vi "Elevator Offset AutoMatic.vi"() -> ()   [LabVIEW 2014]
uses:
  <vilib>/Rock Robotics/WPI/Joystick/WPI_JoystickGetSetRefNum.vi
panel:
  in  "Time Step(ms)":u32=10
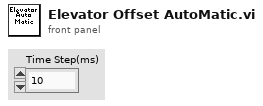
[diagram p1: front panel]
types:
  T1 = typedef "WPI_JoystickDevRef.ctl" = cluster{"Device":T2}
  T2 = typedef "WPI_JoystickDeviceEnum.ctl" = enum16{"USB 0", "USB 1", "USB 2", "USB 3", "USB 4", "USB 5"}
  T3 = typedef "WPI_MotorControlDeviceRef.ctl" = cluster{"DeviceStatus":errorcluster, "Type":T4, "PWM":cluster{"Controller":T5, "PWM Channel":T6, "DeadBand":T7}, "CAN":cluster{"Device Number":u8, "Control Mode":T8, "Semaphore":T9, "Max Vout":dbl, "TalonSRX Control Mode":T10}, "Invert":bool, "TransformRef":T11, "InvTransformRef":T11}
  T4 = typedef "WPI_MotorControlType.ctl" = enum16{"PWM", "CAN", "CANTalonSRX"}
  T5 = typedef "FPGA_TypedefDigitalModule.ctl" = enum16{"Controller 1"}
  T6 = typedef "FPGA_DIOPWMChannel.ctl" = enum8{"PWM 0", "PWM 1", "PWM 2", "PWM 3", "PWM 4", "PWM 5", "PWM 6", "PWM 7", "PWM 8", "PWM 9", "PWM MXP 0", "PWM MXP 1", "PWM MXP 2", "PWM MXP 3", "PWM MXP 4", "PWM MXP 5", "PWM MXP 6", "PWM MXP 7", "PWM MXP 8", "PWM MXP 9", "Invalid"}
  T7 = typedef "WPI_PWMDeadband.ctl" = cluster{"Name":string, "maxPositivePwm":i32, "minPositivePwm":i32, "centerPwm":i32, "maxNegativePwm":i32, "minNegativePwm":i32, "angularRange":u16}
  T8 = typedef "WPI_CANJaguar_ControlMode.ctl" = enum8{"Percent VBus", "Current", "Speed", "Position", "Voltage"}
  T9 = typedef "Semaphore RefNum" = refnum<k1>
  T10 = typedef "WPI_CANTalonSRX_APIControlMode.ctl" = enum8{"Percent VBus", "Speed", "Position", "Slave", "Unchanged / Invalid"}
  T11 = typedef "WPI_PWMTransform_ConPane.ctl" = refnum<vi>
  T12 = typedef "WPI_CANTalonSRX_GlobalStatus.ctl" = cluster{"Applied Throttle":dbl, "Module Enabled":bool, "CAN Error":errorcluster, "Closed Loop Error":dbl, "Forward Limit Switch Closed":bool, "Reverse Limit Switch Closed":bool, "Sensor Position":dbl, "Sensor Velocity":dbl, "Current":dbl, "Sticky Fault - Over Temp":bool, "Sticky Fault - Under Voltage":bool, "Sticky Fault - Forward Limit":bool, "Sticky Fault - Reverse Limit":bool, "Sticky Fault - Forward Soft Limit":bool, "Sticky Fault - Reverse Soft Limit":bool, "Brake is Enabled":bool, "Encoder Position":dbl, "Encoder Velocity":dbl, "Encoder Index Count":dbl, "Encoder A Pin State":bool, "Encoder B Pin State":bool, "Encoder Index Pin State":bool, "Analog In":dbl, "Analog In Velocity":dbl, "Temperature (C)":dbl, "Battery Voltage":dbl}
  T13 = typedef "WPI_SwitchDevRef.ctl" = cluster{"DevStatus":errorcluster, "DIO Channel":T14, "Controller":T5, "CntIndex":T15, "Normally Closed":bool}
  T14 = typedef "FPGA_DIOChannel.ctl" = enum8{"DIO 0", "DIO 1", "DIO 2", "DIO 3", "DIO 4", "DIO 5", "DIO 6", "DIO 7", "DIO 8", "DIO 9", "DIO MXP 0", "DIO MXP 1", "DIO MXP 2", "DIO MXP 3", "DIO MXP 4", "DIO MXP 5", "DIO MXP 6", "DIO MXP 7", "DIO MXP 8", "DIO MXP 9", "DIO MXP 10", "DIO MXP 11", "DIO MXP 12", "DIO MXP 13", "DIO MXP 14", "DIO MXP 15", "Invalid"}
  T15 = typedef "FPGA_CounterCtrSystemIndex.ctl" = enum8{"Ctr 0", "Ctr 1", "Ctr 2", "Ctr 3", "Ctr 4", "Ctr 5", "Ctr 6", "Ctr 7", "Invalid"}
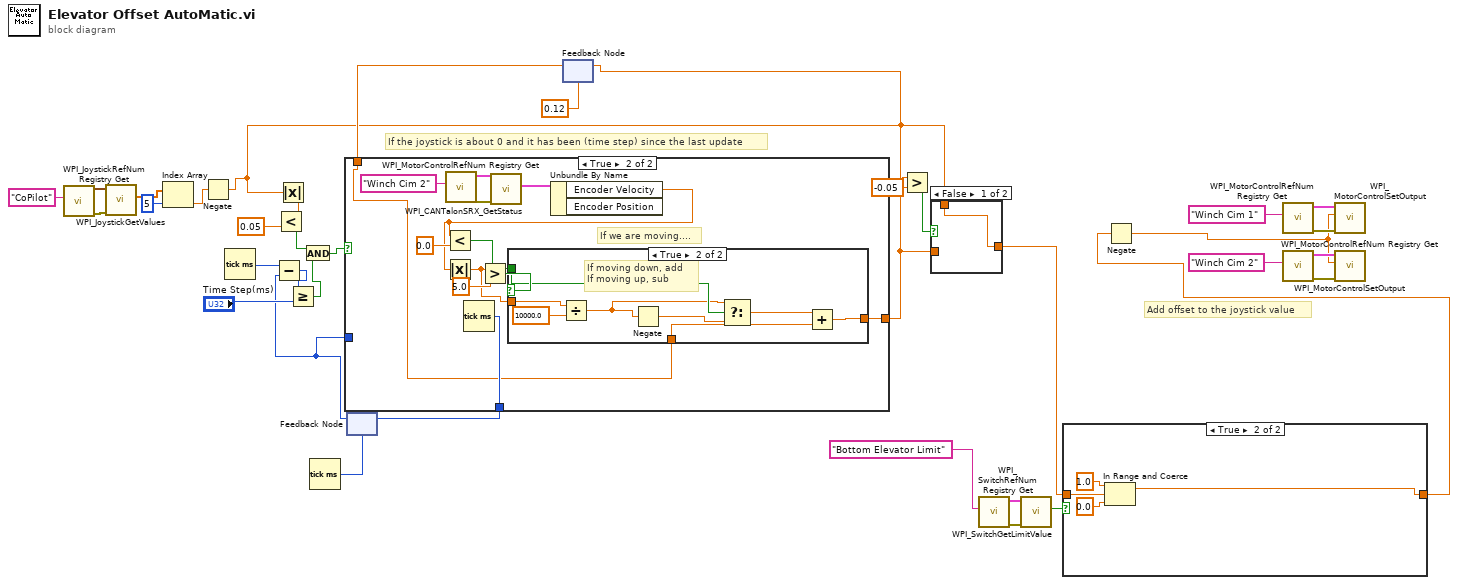
[diagram p0: block diagram]
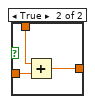
[diagram p2: hidden frame]
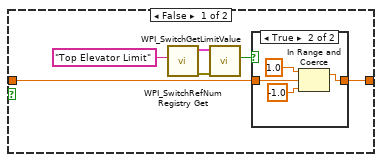
[diagram p3: hidden frame]
diagram:
  # "Add offset to the joystick value"
  # "If the joystick is about 0 and it has been (time step) since the last update"
  n1 = call <vilib>:"WPI_JoystickRefNum Registry Get.vi"("refnum name"="CoPilot") -> ("error out"=w25:errorcluster, "JoystickDevRef"=w26:T1)  [unwired: 9 in]
  n2 = call <vilib>:"WPI_JoystickGetValues.vi"("error in (no error)"=w25, "JoystickDevRef"=w26) -> ("Axes"=w24:dbl[])  [unwired: 5 in, 4 out]
  n3 = Index Array(array=w24, index=5) -> (element=w6:dbl)
  n4 = Negate(x=w6) -> (-x=w2:dbl)
  n5 = Tick Count (ms)() -> (millisecond timer value=w29:u32)
  n6 = Absolute Value(x=w2) -> (abs(x)=w18:dbl)
  n7 = Less?(x=w18, y=0.05) -> (x < y?=w16:bool)
  n8 = Tick Count (ms)() -> (millisecond timer value=w30:u32)
  n9 = feedback #1(w30) -> (w19:u32)
  n10 = Subtract(x=w29, y=w19) -> (x-y=w28:u32)
  n11 = Greater Or Equal?(x=w28, y="Time Step(ms)") -> (x >= y?=w21:bool)
  n12 = And(x=w16, y=w21) -> (x .and. y?=w22:bool)
  n13 = feedback #2(0.12) -> (w14:dbl)
  n14 = case shown="True" w22 {
    tunnel: [w38 w51] -> w20
    tunnel: w19 -> [w38 _]
    tunnel: w14 -> [w37 w46]
    tunnel: [w37 w45] -> w13
    frame False {
    }
    frame True {
      # "If we are moving...."
      n15 = call <vilib>:"WPI_MotorControlRefNum Registry Get.vi"("refnum name"="Winch Cim 2") -> ("error out"=w43:errorcluster, "MotorControlDevRef"=w42:T3)  [unwired: 9 in]
      n16 = Tick Count (ms)() -> (millisecond timer value=w51:u32)
      n17 = call <vilib>:"WPI_CANTalonSRX_GetStatus.vi"("error in (no error)"=w43, "CAN Talon SRX Ref"=w42) -> ("Talon SRX Status"=w41:T12)  [unwired: 7 in, 2 out]
      n18 = Unbundle By Name(w41) -> ("Encoder Velocity"=w40:dbl)  [unwired: 1 out]
      n19 = Less?(x=w40, y=0.0) -> (x < y?=w47:bool)
      n20 = Absolute Value(x=w40) -> (abs(x)=w39:dbl)
      n21 = Greater?(x=w39, y=5.0) -> (0:w48:bool)
      n22 = case shown="True" w48 {
        tunnel: w47 -> [_ w60]
        tunnel: w46 -> [w52 w58]
        tunnel: [w52 w57] -> w45
        tunnel: w39 -> [_ w55]
        frame False {
        }
        frame True {
          # "If moving down, add\nIf moving up, sub"
          n23 = Divide(x=w55, y=10000.0) -> (x/y=w53:dbl)
          n24 = Negate(x=w53) -> (-x=w54:dbl)
          n25 = Select(t=w53, s=w60, f=w54) -> (s? t:f=w59:dbl)
          n26 = Add(x=w59, y=w58) -> (x+y=w57:dbl)
        }
      }
    }
  }
  n27 = feedback-in #1(w20) -> ()
  n28 = feedback-in #2(w13) -> ()
  n29 = Greater?(x=w2, y=-0.05) -> (0:w1:bool)
  n30 = case shown="False" w1 {
    tunnel: w13 -> [_ w64]
    tunnel: [w61 w63] -> w8
    tunnel: w2 -> [w61 w62]
    frame False {
    }
    frame True {
      n31 = Add(x=w62, y=w64) -> (x+y=w63:dbl)
    }
  }
  n32 = call <vilib>:"WPI_SwitchRefNum Registry Get.vi"("refnum name"="Bottom Elevator Limit") -> ("error out"=w12:errorcluster, "SwitchDevRef"=w11:T13)  [unwired: 9 in]
  n33 = call <vilib>:"WPI_SwitchGetLimitValue.vi"("error in (no error)"=w12, "SwitchDevRef"=w11) -> ("Switch Pressed"=w10:bool)  [unwired: 7 in, 2 out]
  n34 = case shown="True" w10 {
    tunnel: w8 -> [w70 w77]
    tunnel: [w69 w76] -> w7
    frame False {
      n35 = call <vilib>:"WPI_SwitchRefNum Registry Get.vi"("refnum name"="Top Elevator Limit") -> ("error out"=w68:errorcluster, "SwitchDevRef"=w67:T13)  [unwired: 9 in]
      n36 = call <vilib>:"WPI_SwitchGetLimitValue.vi"("error in (no error)"=w68, "SwitchDevRef"=w67) -> ("Switch Pressed"=w65:bool)  [unwired: 7 in, 2 out]
      n37 = case shown="True" w65 {
        tunnel: w70 -> [w71 w73]
        tunnel: [w71 w72] -> w69
        frame False {
        }
        frame True {
          n38 = In Range and Coerce(upper limit=1.0, x=w73, lower limit=-1.0) -> (coerced(x)=w72:dbl)  [unwired: 1 out]
        }
      }
    }
    frame True {
      n39 = In Range and Coerce(upper limit=1.0, x=w77, lower limit=0.0) -> (coerced(x)=w76:dbl)  [unwired: 1 out]
    }
  }
  n40 = Negate(x=w7) -> (-x=w5:dbl)
  n41 = call <vilib>:"WPI_MotorControlRefNum Registry Get.vi"("refnum name"="Winch Cim 1") -> ("error out"=w36:errorcluster, "MotorControlDevRef"=w35:T3)  [unwired: 9 in]
  n42 = call <vilib>:"WPI_MotorControlRefNum Registry Get.vi"("refnum name"="Winch Cim 2") -> ("error out"=w33:errorcluster, "MotorControlDevRef"=w32:T3)  [unwired: 9 in]
  n43 = call <vilib>:"WPI_MotorControlSetOutput.vi"("error in (no error)"=w36, "Output"=w5, "MotorControlDevRef"=w35) -> ()  [unwired: 6 in, 3 out]
  n44 = call <vilib>:"WPI_MotorControlSetOutput.vi"("error in (no error)"=w33, "Output"=w5, "MotorControlDevRef"=w32) -> ()  [unwired: 6 in, 3 out]
